vi "Uptime Monitor (SubVI).vi"(7 "Queue in":refnum<queue>, 11 "Start ms":u32) -> (3 "Uptime String":string)   [LabVIEW 2019]
uses:
  Globals and Definitions/System Message.ctl
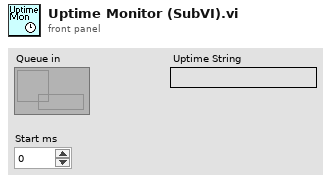
[diagram p1: front panel]
types:
  T1 = typedef "System Message.ctl" = cluster{"Message Tag":string, "Message Body":string, "Snooze Time (s)":dbl, "Snooze Alert?":bool, "Log Event?":bool, "Send Email":i32}
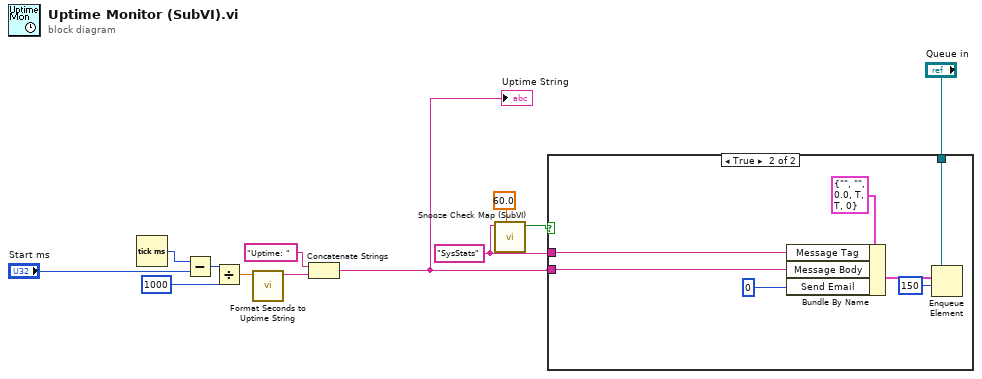
[diagram p0: block diagram]
diagram:
  w8 = "SysStats" ("Message Tag")
  n1 = Tick Count (ms)() -> (millisecond timer value=w3:u32)
  n2 = Subtract(x=w3, y="Start ms") -> (x-y=w4:u32)
  n3 = Divide(x=w4, y=u32 1000) -> (x/y=w6:dbl)
  n4 = call "Format Seconds to Uptime String.vi"("Elapsed Time (s)"=w6) -> ("Uptime String"=w7:string)  [unwired: 10 in]
  n5 = Concatenate Strings("Uptime: " ("string"), w7) -> (w12:string)
  "Uptime String" <- w12
  n6 = call "Snooze Check Map (SubVI).vi"("Snooze Time (s)"=60.0, "key"=w8) -> ("Snooze Expired?"=w9:bool)  [unwired: 9 in]
  n7 = case shown="True" w9 {
    tunnel: w8 -> [_ w16]
    tunnel: w12 -> [_ w14]
    tunnel: "Queue in" -> [_ w15]
    frame False {
    }
    frame True {
      n8 = Bundle By Name(cluster=T1 {"Message Tag"="", "Message Body"="", "Snooze Time (s)"=0.0, "Snooze Alert?"=TRUE, "Log Event?"=TRUE, "Send Email"=0}, "Message Tag"=w16, "Message Body"=w14, "Send Email"=0) -> (w17:T1)
      n9 = Enqueue Element(queue=w15, element=w17, timeout in ms (-1)=150) -> ()  [unwired: 1 in, 3 out]
    }
  }
